vi "Merge Two Structures.vi"(9 "Translation Vector (1 to 2)":dbl[](array[numeric])=[0.0, 0.0, 17.5617], 10 "Atomic Structure 2":T1={"Structure Name"="Batch6_1", "Lattice vector a"=[9.1641, 0.0, 0.0], "Lattice vector b"=[0.0, 7.93635, 0.0], "Lattice vector c"=[0.0, 0.0, 17.5617], "Atoms Array"=[{"Atom Name"="Cd", "Positions (Direct)"=[[1e-06, 0.133333, 0.072927], [0.500001, 0.133333, 0.072927], [0.250001, 0.633333, 0.072927], [0.750001, 0.633333, 0.072927], [0.250001, 0.3, 0.285961], [0.750001, 0.3, 0.285961], [1e-06, 0.8, 0.285961], [0.500001, 0.8, 0.285961], [1e-06, 0.466667, 0.498995], [0.500001, 0.466667, 0.498995], [0.250001, 0.966667, 0.498995], [0.750001, 0.966667, 0.498995], [0.25, 0.134593, 0.662792], [0.75, 0.134593, 0.662792], [0.0, 0.634593, 0.662792], [0.5, 0.634593, 0.662792], [0.125, 0.467068, 0.873815], [0.625, 0.467068, 0.873815], [0.375, 0.967067, 0.873815], [0.875, 0.967067, 0.873815]], "Positions (Cartesian)"=[[9.1641e-06, 1.05817735455, 1.2807220959], [4.5820591641, 1.05817735455, 1.2807220959], [2.2910341640999996, 5.02635235455, 1.2807220959], [6.8730841641, 5.02635235455, 1.2807220959], [2.2910341640999996, 2.380905, 5.0219612936999996], [6.8730841641, 2.380905, 5.0219612936999996], [9.1641e-06, 6.349080000000001, 5.0219612936999996], [4.5820591641, 6.349080000000001, 5.0219612936999996], [9.1641e-06, 3.70363264545, 8.7632004915], [4.5820591641, 3.70363264545, 8.7632004915], [2.2910341640999996, 7.67180764545, 8.7632004915], [6.8730841641, 7.67180764545, 8.7632004915], [2.291025, 1.06817715555, 11.639754266399999], [6.873075, 1.06817715555, 11.639754266399999], [0.0, 5.0363521555499995, 11.639754266399999], [4.58205, 5.0363521555499995, 11.639754266399999], [1.1455125, 3.7068151218, 15.345676885499998], [5.7275624999999994, 3.7068151218, 15.345676885499998], [3.4365375, 7.67498218545, 15.345676885499998], [8.018587499999999, 7.67498218545, 15.345676885499998]]}, {"Atom Name"="Te", "Positions (Direct)"=[[0.250001, 0.3, 0.126185], [0.750001, 0.3, 0.126185], [1e-06, 0.8, 0.126185], [0.500001, 0.8, 0.126185], [1e-06, 0.466667, 0.339219], [0.500001, 0.466667, 0.339219], [0.250001, 0.966667, 0.339219], [0.750001, 0.966667, 0.339219], [1e-06, 0.133333, 0.552254], [0.500001, 0.133333, 0.552254], [0.250001, 0.633333, 0.552254], [0.750001, 0.633333, 0.552254], [0.25, 0.467926, 0.71605], [0.75, 0.467926, 0.71605], [0.0, 0.967926, 0.71605], [0.5, 0.967926, 0.71605], [0.125, 0.133735, 0.927073], [0.625, 0.133735, 0.927073], [0.375, 0.633734, 0.927073], [0.875, 0.633734, 0.927073]], "Positions (Cartesian)"=[[2.2910341640999996, 2.380905, 2.2160231144999996], [6.8730841641, 2.380905, 2.2160231144999996], [9.1641e-06, 6.349080000000001, 2.2160231144999996], [4.5820591641, 6.349080000000001, 2.2160231144999996], [9.1641e-06, 3.70363264545, 5.957262312299999], [4.5820591641, 3.70363264545, 5.957262312299999], [2.2910341640999996, 7.67180764545, 5.957262312299999], [6.8730841641, 7.67180764545, 5.957262312299999], [9.1641e-06, 1.05817735455, 9.6985190718], [4.5820591641, 1.05817735455, 9.6985190718], [2.2910341640999996, 5.02635235455, 9.6985190718], [6.8730841641, 5.02635235455, 9.6985190718], [2.291025, 3.7136245101000003, 12.575055284999998], [6.873075, 3.7136245101000003, 12.575055284999998], [0.0, 7.681799510099999, 12.575055284999998], [4.58205, 7.681799510099999, 12.575055284999998], [1.1455125, 1.06136776725, 16.2809779041], [5.7275624999999994, 1.06136776725, 16.2809779041], [3.4365375, 5.0295348309, 16.2809779041], [8.018587499999999, 5.0295348309, 16.2809779041]]}], "# of atoms"=40}, 11 "Atomic Structure 1":T1={"Structure Name"="Batch6_1", "Lattice vector a"=[9.1641, 0.0, 0.0], "Lattice vector b"=[0.0, 7.93635, 0.0], "Lattice vector c"=[0.0, 0.0, 17.5617], "Atoms Array"=[{"Atom Name"="Cd", "Positions (Direct)"=[[1e-06, 0.133333, 0.072927], [0.500001, 0.133333, 0.072927], [0.250001, 0.633333, 0.072927], [0.750001, 0.633333, 0.072927], [0.250001, 0.3, 0.285961], [0.750001, 0.3, 0.285961], [1e-06, 0.8, 0.285961], [0.500001, 0.8, 0.285961], [1e-06, 0.466667, 0.498995], [0.500001, 0.466667, 0.498995], [0.250001, 0.966667, 0.498995], [0.750001, 0.966667, 0.498995], [0.25, 0.134593, 0.662792], [0.75, 0.134593, 0.662792], [0.0, 0.634593, 0.662792], [0.5, 0.634593, 0.662792], [0.125, 0.467068, 0.873815], [0.625, 0.467068, 0.873815], [0.375, 0.967067, 0.873815], [0.875, 0.967067, 0.873815]], "Positions (Cartesian)"=[[9.1641e-06, 1.05817735455, 1.2807220959], [4.5820591641, 1.05817735455, 1.2807220959], [2.2910341640999996, 5.02635235455, 1.2807220959], [6.8730841641, 5.02635235455, 1.2807220959], [2.2910341640999996, 2.380905, 5.0219612936999996], [6.8730841641, 2.380905, 5.0219612936999996], [9.1641e-06, 6.349080000000001, 5.0219612936999996], [4.5820591641, 6.349080000000001, 5.0219612936999996], [9.1641e-06, 3.70363264545, 8.7632004915], [4.5820591641, 3.70363264545, 8.7632004915], [2.2910341640999996, 7.67180764545, 8.7632004915], [6.8730841641, 7.67180764545, 8.7632004915], [2.291025, 1.06817715555, 11.639754266399999], [6.873075, 1.06817715555, 11.639754266399999], [0.0, 5.0363521555499995, 11.639754266399999], [4.58205, 5.0363521555499995, 11.639754266399999], [1.1455125, 3.7068151218, 15.345676885499998], [5.7275624999999994, 3.7068151218, 15.345676885499998], [3.4365375, 7.67498218545, 15.345676885499998], [8.018587499999999, 7.67498218545, 15.345676885499998]]}, {"Atom Name"="Te", "Positions (Direct)"=[[0.250001, 0.3, 0.126185], [0.750001, 0.3, 0.126185], [1e-06, 0.8, 0.126185], [0.500001, 0.8, 0.126185], [1e-06, 0.466667, 0.339219], [0.500001, 0.466667, 0.339219], [0.250001, 0.966667, 0.339219], [0.750001, 0.966667, 0.339219], [1e-06, 0.133333, 0.552254], [0.500001, 0.133333, 0.552254], [0.250001, 0.633333, 0.552254], [0.750001, 0.633333, 0.552254], [0.25, 0.467926, 0.71605], [0.75, 0.467926, 0.71605], [0.0, 0.967926, 0.71605], [0.5, 0.967926, 0.71605], [0.125, 0.133735, 0.927073], [0.625, 0.133735, 0.927073], [0.375, 0.633734, 0.927073], [0.875, 0.633734, 0.927073]], "Positions (Cartesian)"=[[2.2910341640999996, 2.380905, 2.2160231144999996], [6.8730841641, 2.380905, 2.2160231144999996], [9.1641e-06, 6.349080000000001, 2.2160231144999996], [4.5820591641, 6.349080000000001, 2.2160231144999996], [9.1641e-06, 3.70363264545, 5.957262312299999], [4.5820591641, 3.70363264545, 5.957262312299999], [2.2910341640999996, 7.67180764545, 5.957262312299999], [6.8730841641, 7.67180764545, 5.957262312299999], [9.1641e-06, 1.05817735455, 9.6985190718], [4.5820591641, 1.05817735455, 9.6985190718], [2.2910341640999996, 5.02635235455, 9.6985190718], [6.8730841641, 5.02635235455, 9.6985190718], [2.291025, 3.7136245101000003, 12.575055284999998], [6.873075, 3.7136245101000003, 12.575055284999998], [0.0, 7.681799510099999, 12.575055284999998], [4.58205, 7.681799510099999, 12.575055284999998], [1.1455125, 1.06136776725, 16.2809779041], [5.7275624999999994, 1.06136776725, 16.2809779041], [3.4365375, 5.0295348309, 16.2809779041], [8.018587499999999, 5.0295348309, 16.2809779041]]}], "# of atoms"=40}) -> (3 "Atomic Structure of 1 + 2 by T":T1={"Structure Name"="Batch6_1+Batch6_1", "Lattice vector a"=[9.1641, 0.0, 0.0], "Lattice vector b"=[0.0, 7.93635, 0.0], "Lattice vector c"=[0.0, 0.0, 35.1234], "Atoms Array"=[{"Atom Name"="Cd", "Positions (Direct)"=[[1e-06, 0.13333299999999998, 0.03646350000000001], [0.500001, 0.13333299999999998, 0.03646350000000001], [0.250001, 0.6333329999999999, 0.03646350000000001], [0.750001, 0.6333329999999999, 0.03646350000000001], [0.250001, 0.29999999999999993, 0.1429805], [0.750001, 0.29999999999999993, 0.1429805], [1e-06, 0.8, 0.1429805], [0.500001, 0.8, 0.1429805], [1e-06, 0.46666699999999994, 0.2494975], [0.500001, 0.46666699999999994, 0.2494975], [0.250001, 0.9666669999999999, 0.2494975], [0.750001, 0.9666669999999999, 0.2494975], [0.25, 0.134593, 0.331396], [0.75, 0.134593, 0.331396], [0.0, 0.6345929999999999, 0.331396], [0.5, 0.6345929999999999, 0.331396], [0.125, 0.467068, 0.4369075], [0.625, 0.467068, 0.4369075], [0.375, 0.9670669999999999, 0.4369075], [0.8749999999999999, 0.9670669999999999, 0.4369075], [1e-06, 0.13333299999999998, 0.5364635], [0.500001, 0.13333299999999998, 0.5364635], [0.250001, 0.6333329999999999, 0.5364635], [0.750001, 0.6333329999999999, 0.5364635], [0.250001, 0.29999999999999993, 0.6429805], [0.750001, 0.29999999999999993, 0.6429805], [1e-06, 0.8, 0.6429805], [0.500001, 0.8, 0.6429805], [1e-06, 0.46666699999999994, 0.7494974999999999], [0.500001, 0.46666699999999994, 0.7494974999999999], [0.250001, 0.9666669999999999, 0.7494974999999999], [0.750001, 0.9666669999999999, 0.7494974999999999], [0.25, 0.134593, 0.831396], [0.75, 0.134593, 0.831396], [0.0, 0.6345929999999999, 0.831396], [0.5, 0.6345929999999999, 0.831396], [0.125, 0.467068, 0.9369075000000001], [0.625, 0.467068, 0.9369075000000001], [0.375, 0.9670669999999999, 0.9369075000000001], [0.8749999999999999, 0.9670669999999999, 0.9369075000000001]], "Positions (Cartesian)"=[[9.1641e-06, 1.05817735455, 1.2807220959], [4.5820591641, 1.05817735455, 1.2807220959], [2.2910341640999996, 5.02635235455, 1.2807220959], [6.8730841641, 5.02635235455, 1.2807220959], [2.2910341640999996, 2.380905, 5.0219612936999996], [6.8730841641, 2.380905, 5.0219612936999996], [9.1641e-06, 6.349080000000001, 5.0219612936999996], [4.5820591641, 6.349080000000001, 5.0219612936999996], [9.1641e-06, 3.70363264545, 8.7632004915], [4.5820591641, 3.70363264545, 8.7632004915], [2.2910341640999996, 7.67180764545, 8.7632004915], [6.8730841641, 7.67180764545, 8.7632004915], [2.291025, 1.06817715555, 11.639754266399999], [6.873075, 1.06817715555, 11.639754266399999], [0.0, 5.0363521555499995, 11.639754266399999], [4.58205, 5.0363521555499995, 11.639754266399999], [1.1455125, 3.7068151218, 15.345676885499998], [5.7275624999999994, 3.7068151218, 15.345676885499998], [3.4365375, 7.67498218545, 15.345676885499998], [8.018587499999999, 7.67498218545, 15.345676885499998], [9.1641e-06, 1.05817735455, 18.842422095899998], [4.5820591641, 1.05817735455, 18.842422095899998], [2.2910341640999996, 5.02635235455, 18.842422095899998], [6.8730841641, 5.02635235455, 18.842422095899998], [2.2910341640999996, 2.380905, 22.583661293699997], [6.8730841641, 2.380905, 22.583661293699997], [9.1641e-06, 6.349080000000001, 22.583661293699997], [4.5820591641, 6.349080000000001, 22.583661293699997], [9.1641e-06, 3.70363264545, 26.324900491499996], [4.5820591641, 3.70363264545, 26.324900491499996], [2.2910341640999996, 7.67180764545, 26.324900491499996], [6.8730841641, 7.67180764545, 26.324900491499996], [2.291025, 1.06817715555, 29.2014542664], [6.873075, 1.06817715555, 29.2014542664], [0.0, 5.0363521555499995, 29.2014542664], [4.58205, 5.0363521555499995, 29.2014542664], [1.1455125, 3.7068151218, 32.9073768855], [5.7275624999999994, 3.7068151218, 32.9073768855], [3.4365375, 7.67498218545, 32.9073768855], [8.018587499999999, 7.67498218545, 32.9073768855]]}, {"Atom Name"="Te", "Positions (Direct)"=[[0.250001, 0.29999999999999993, 0.0630925], [0.750001, 0.29999999999999993, 0.0630925], [1e-06, 0.8, 0.0630925], [0.500001, 0.8, 0.0630925], [1e-06, 0.46666699999999994, 0.1696095], [0.500001, 0.46666699999999994, 0.1696095], [0.250001, 0.9666669999999999, 0.1696095], [0.750001, 0.9666669999999999, 0.1696095], [1e-06, 0.13333299999999998, 0.276127], [0.500001, 0.13333299999999998, 0.276127], [0.250001, 0.6333329999999999, 0.276127], [0.750001, 0.6333329999999999, 0.276127], [0.25, 0.467926, 0.358025], [0.75, 0.467926, 0.358025], [0.0, 0.9679259999999998, 0.358025], [0.5, 0.9679259999999998, 0.358025], [0.125, 0.133735, 0.4635365], [0.625, 0.133735, 0.4635365], [0.375, 0.633734, 0.4635365], [0.8749999999999999, 0.633734, 0.4635365], [0.250001, 0.29999999999999993, 0.5630925], [0.750001, 0.29999999999999993, 0.5630925], [1e-06, 0.8, 0.5630925], [0.500001, 0.8, 0.5630925], [1e-06, 0.46666699999999994, 0.6696095], [0.500001, 0.46666699999999994, 0.6696095], [0.250001, 0.9666669999999999, 0.6696095], [0.750001, 0.9666669999999999, 0.6696095], [1e-06, 0.13333299999999998, 0.776127], [0.500001, 0.13333299999999998, 0.776127], [0.250001, 0.6333329999999999, 0.776127], [0.750001, 0.6333329999999999, 0.776127], [0.25, 0.467926, 0.858025], [0.75, 0.467926, 0.858025], [0.0, 0.9679259999999998, 0.858025], [0.5, 0.9679259999999998, 0.858025], [0.125, 0.133735, 0.9635365000000001], [0.625, 0.133735, 0.9635365000000001], [0.375, 0.633734, 0.9635365000000001], [0.8749999999999999, 0.633734, 0.9635365000000001]], "Positions (Cartesian)"=[[2.2910341640999996, 2.380905, 2.2160231144999996], [6.8730841641, 2.380905, 2.2160231144999996], [9.1641e-06, 6.349080000000001, 2.2160231144999996], [4.5820591641, 6.349080000000001, 2.2160231144999996], [9.1641e-06, 3.70363264545, 5.957262312299999], [4.5820591641, 3.70363264545, 5.957262312299999], [2.2910341640999996, 7.67180764545, 5.957262312299999], [6.8730841641, 7.67180764545, 5.957262312299999], [9.1641e-06, 1.05817735455, 9.6985190718], [4.5820591641, 1.05817735455, 9.6985190718], [2.2910341640999996, 5.02635235455, 9.6985190718], [6.8730841641, 5.02635235455, 9.6985190718], [2.291025, 3.7136245101000003, 12.575055284999998], [6.873075, 3.7136245101000003, 12.575055284999998], [0.0, 7.681799510099999, 12.575055284999998], [4.58205, 7.681799510099999, 12.575055284999998], [1.1455125, 1.06136776725, 16.2809779041], [5.7275624999999994, 1.06136776725, 16.2809779041], [3.4365375, 5.0295348309, 16.2809779041], [8.018587499999999, 5.0295348309, 16.2809779041], [2.2910341640999996, 2.380905, 19.7777231145], [6.8730841641, 2.380905, 19.7777231145], [9.1641e-06, 6.349080000000001, 19.7777231145], [4.5820591641, 6.349080000000001, 19.7777231145], [9.1641e-06, 3.70363264545, 23.518962312299998], [4.5820591641, 3.70363264545, 23.518962312299998], [2.2910341640999996, 7.67180764545, 23.518962312299998], [6.8730841641, 7.67180764545, 23.518962312299998], [9.1641e-06, 1.05817735455, 27.260219071799998], [4.5820591641, 1.05817735455, 27.260219071799998], [2.2910341640999996, 5.02635235455, 27.260219071799998], [6.8730841641, 5.02635235455, 27.260219071799998], [2.291025, 3.7136245101000003, 30.136755284999996], [6.873075, 3.7136245101000003, 30.136755284999996], [0.0, 7.681799510099999, 30.136755284999996], [4.58205, 7.681799510099999, 30.136755284999996], [1.1455125, 1.06136776725, 33.8426779041], [5.7275624999999994, 1.06136776725, 33.8426779041], [3.4365375, 5.0295348309, 33.8426779041], [8.018587499999999, 5.0295348309, 33.8426779041]]}], "# of atoms"=80})   [LabVIEW 2010]
uses:
  <vilib>/Analysis/baseanly.llb/Real Inverse Matrix.vi
  <vilib>/Analysis/baseanly.llb/A x Vector.vi
  <vilib>/Analysis/NI_AALBase.lvlib
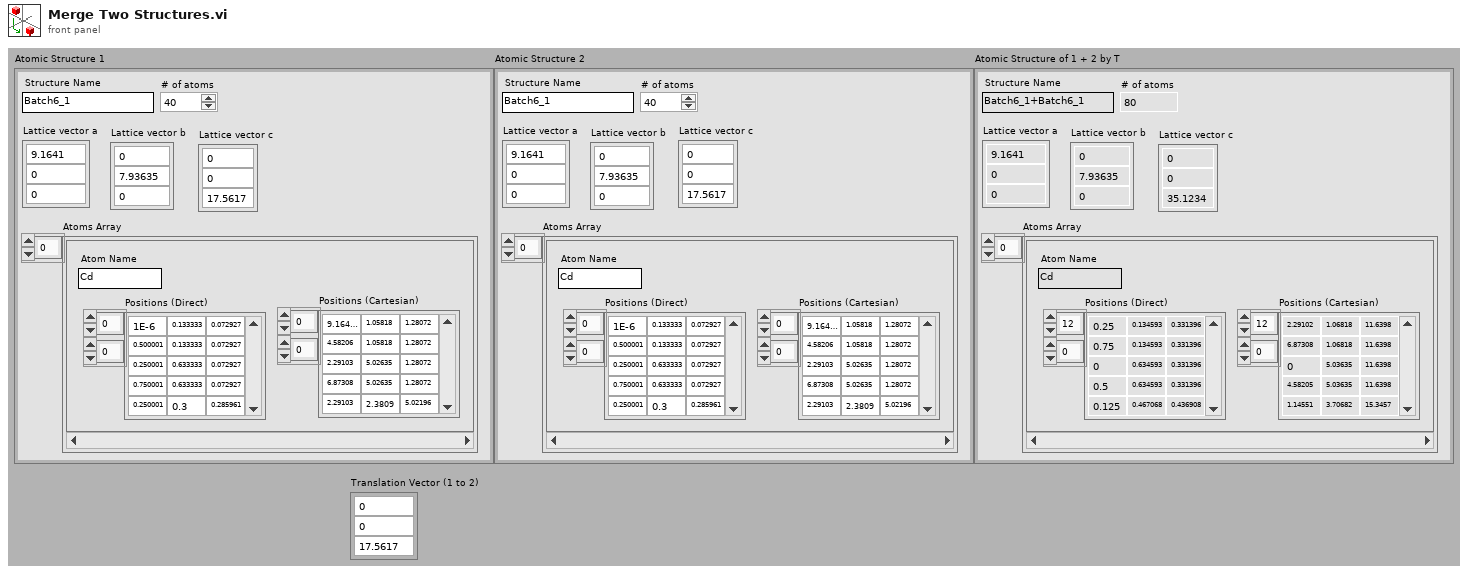
[diagram p1: front panel]
types:
  T1 = cluster{"Structure Name":string, "Lattice vector a":dbl[], "Lattice vector b":dbl[], "Lattice vector c":dbl[], "Atoms Array":cluster{"Atom Name":string, "Positions (Direct)":dbl[][], "Positions (Cartesian)":dbl[][]}[], "# of atoms":i32}
  T2 = cluster{"Atom Name":string, "Positions (Direct)":dbl[][], "Positions (Cartesian)":dbl[][]}[]
  T3 = typedef "NI_Matrix.lvlib/RealMatrix.ctl" = dbl[][]
  T4 = cluster{string, dbl[], dbl[], dbl[], cluster{"Atom Name":string, dbl[][], dbl[][]}[], i32}
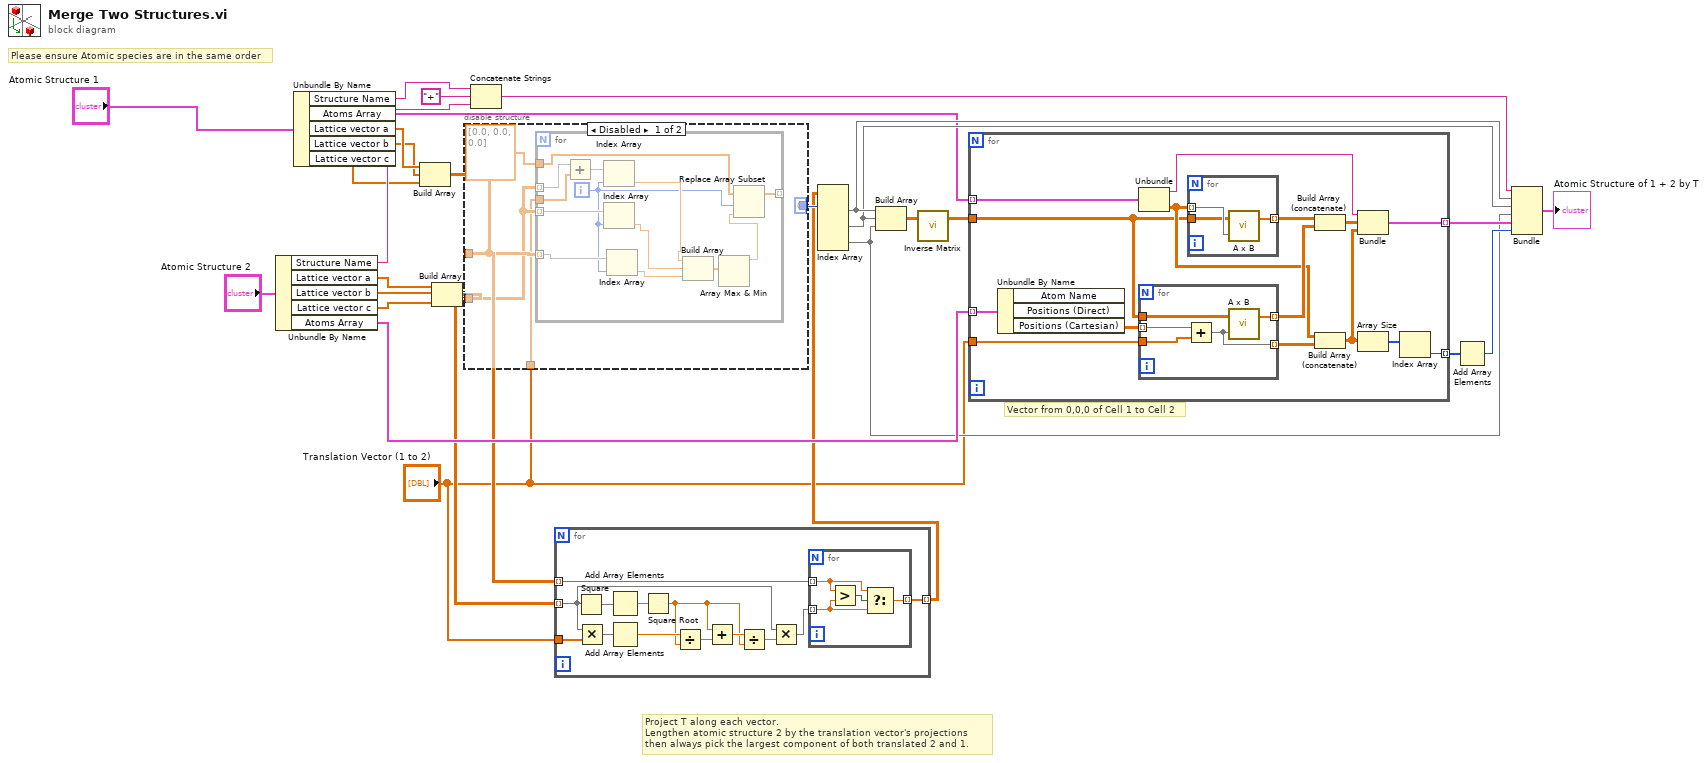
[diagram p0: block diagram]
diagram:
  # "Project T along each vector.\nLengthen atomic structure 2 by the translation vector's projections\nthen always pick the largest component of both translated 2 and 1."
  # "Please ensure Atomic species are in the same order"
  # "Vector from 0,0,0 of Cell 1 to Cell 2"
  n1 = Unbundle By Name("Atomic Structure 2") -> ("Structure Name"=w16:string, "Lattice vector a"=w25:dbl[], "Lattice vector b"=w24:dbl[], "Lattice vector c"=w23:dbl[], "Atoms Array"=w27:T2)
  n2 = Unbundle By Name("Atomic Structure 1") -> ("Structure Name"=w18:string, "Atoms Array"=w8:T2, "Lattice vector a"=w7:dbl[], "Lattice vector b"=w6:dbl[], "Lattice vector c"=w5:dbl[])
  n3 = Build Array(w7, w6, w5) -> (w4:dbl[][])
  n4 = Build Array(w25, w24, w23) -> (w3:dbl[][])
  n5 = disable-structure shown="Disabled" {
    disable-tunnel: [0 ("index (row)") _] -> w22
    disable-tunnel: w4 -> [w31 _]
    disable-tunnel: w3 -> [w30 _]
    disable-tunnel: "Translation Vector (1 to 2)" -> [w29 _]
    frame Disabled {
      n6 = for {
        tunnel: w30 -> [w46] mode=indexing
        tunnel: w30 -> [w45] mode=indexing
        tunnel: w29 -> [w44]
        tunnel: dbl[] [0.0, 0.0, 0.0] ("appended array") -> [w42]
        tunnel: [w41] -> _ mode=indexing
        tunnel: w31 -> [w40] mode=indexing
        i -> [w34]
        n7 = Add(x=w45, y=w44) -> (x+y=w43:dbl[])
        n8 = Index Array(array=w43, index=w34) -> (element=w37:dbl)
        n9 = Index Array(array=w46, index=w34) -> (element=w38:dbl)
        n10 = Index Array(array=w40, index=w34) -> (element=w39:dbl)
        n11 = Build Array(w37, w38, w39) -> (w36:dbl[])
        n12 = Array Max & Min(array=w36) -> (max value=w35:dbl)  [unwired: 3 out]
        n13 = Replace Array Subset(array=w42, new element=w35, index=w34) -> (w41:dbl[])
      }
    }
    frame Enabled {
    }
  }
  n14 = Concatenate Strings(w18, "+" ("string"), w16) -> (w15:string)
  n15 = for {
    tunnel: w4 -> [w48] mode=indexing
    tunnel: w3 -> [w50] mode=indexing
    tunnel: [w47] -> w2 mode=indexing
    tunnel: "Translation Vector (1 to 2)" -> [w59]
    n16 = Square(x=w50) -> (x^2=w57:dbl[])
    n17 = Multiply(x=w50, y=w59) -> (x*y=w58:dbl[])
    n18 = Add Array Elements(numeric array=w57) -> (sum=w56:dbl)
    n19 = Add Array Elements(numeric array=w58) -> (sum=w55:dbl)
    n20 = Square Root(x=w56) -> (sqrt(x)=w52:dbl)
    n21 = Divide(x=w55, y=w52) -> (x/y=w54:dbl)
    n22 = Add(x=w52, y=w54) -> (x+y=w53:dbl)
    n23 = Divide(x=w53, y=w52) -> (x/y=w51:dbl)
    n24 = Multiply(x=w50, y=w51) -> (x*y=w49:dbl[])
    n25 = for {
      tunnel: w49 -> [w61] mode=indexing
      tunnel: w48 -> [w62] mode=indexing
      tunnel: [w60] -> w47 mode=indexing
      n26 = Greater?(x=w62, y=w61) -> (0:w63:bool)
      n27 = Select(t=w62, s=w63, f=w61) -> (s? t:f=w60:dbl)
    }
  }
  n28 = Index Array(array=w2, index (row) #1=w22) -> (element #1=w13:dbl[], element #2=w12:dbl[], element #3=w11:dbl[])  [unwired: 5 in]
  n29 = Build Array(w13, w12, w11) -> (w10:T3)
  n30 = call-poly <vilib>:"Inverse Matrix.vi"("Input Matrix"=w10) -> ("Inverse Matrix"=w9:T3)  [unwired: 1 in, 1 out]
  n31 = for {
    tunnel: w27 -> [w78] mode=indexing
    tunnel: "Translation Vector (1 to 2)" -> [w75]
    tunnel: w8 -> [w77] mode=indexing
    tunnel: [w71] -> w21 mode=indexing
    tunnel: [w69] -> w20 mode=indexing
    tunnel: w9 -> [w64]
    n32 = Unbundle By Name(w78) -> ("Positions (Cartesian)"=w76:dbl[][])  [unwired: 2 out]
    n33 = Unbundle(w77) -> ("Atom Name"=w73:string, "Positions (Cartesian)"=w66:dbl[][])  [unwired: 1 out]
    n34 = for {
      tunnel: w76 -> [w86] mode=indexing
      tunnel: w75 -> [w85]
      tunnel: [w83] -> w74 mode=indexing
      tunnel: w64 -> [w84]
      tunnel: [w82] -> w68 mode=indexing
      n35 = Add(x=w86, y=w85) -> (x+y=w83:dbl[])
      n36 = call-poly <vilib>:"A x B.vi"("Vector"=w83, "A"=w84) -> ("A x Vector"=w82:dbl[])  [unwired: 1 out]
    }
    n37 = for {
      tunnel: w66 -> [w81] mode=indexing
      tunnel: [w80] -> w65 mode=indexing
      tunnel: w64 -> [w79]
      n38 = call-poly <vilib>:"A x B.vi"("Vector"=w81, "A"=w79) -> ("A x Vector"=w80:dbl[])  [unwired: 1 out]
    }
    n39 = Build Array (concatenate)(w65, w68) -> (w67:dbl[][])
    n40 = Build Array (concatenate)(w66, w74) -> (w70:dbl[][])
    n41 = Bundle("Atom Name"=w73, w67, w70) -> (w69:cluster{"Atom Name":string, dbl[][], dbl[][]})  [unwired: 1 in]
    n42 = Array Size(array=w70) -> (size(s)=w72:i32[])
    n43 = Index Array(array=w72) -> (element=w71:i32)  [unwired: 1 in]
  }
  n44 = Add Array Elements(numeric array=w21) -> (sum=w19:i32)
  n45 = Bundle(w15, w13, w12, w11, w20, w19) -> (→"Atomic Structure of 1 + 2 by T":T4)  [unwired: 1 in]
